vi "VI Server_GetClusterControlRefsAndMergeWithMainDataCluster.vi"(7 "Cluster.LabelArray":string[](array[string]), 8 "error in":errorcluster, 11 "VI Server Cluster":T1) -> (0 "error out":errorcluster, 1 "Cluster.ControRefs":refnum<vi>[](array[refnum]), 2 "Cluster.ControlLabels":string[](array[string]), 3 "VI Server Cluster.OUT":T1)   [LabVIEW 2020]
doc: "Retrieves multiple clusters' content labels and associated references and adds them to VI Server Cluster.\nIn addition it returns arrays of references and labels of the specified clusters.\n\nThis way these controls can be accessed via VI Server Tools.\nPlease keep in mind the labels should be unique in order to be properly identified."
uses:
  VI Server_TypeDefs/VI Server_RefsCluster.ctl
  VI Server Toolkit LV2013.lvlib
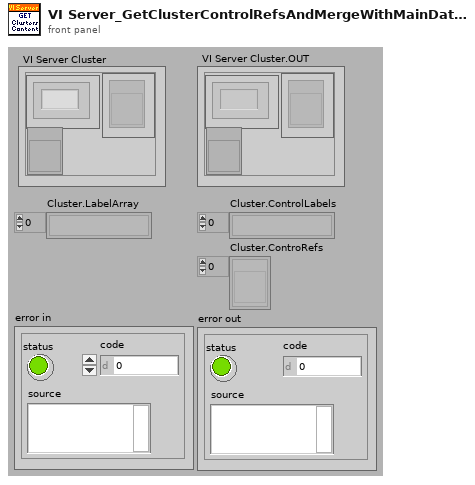
[diagram p1: front panel]
types:
  T1 = typedef "VI Server_RefsCluster.ctl" = cluster{"Labels":string[], "Refs":refnum<vi>[], "VI Ref":refnum<vi>}
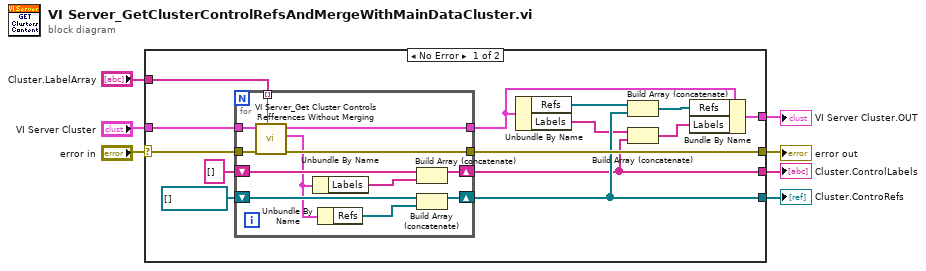
[diagram p0: block diagram]
diagram:
  n1 = case shown="No Error" "error in" {
    selector: "error in" -> [w16 w34]
    tunnel: [w11 _] -> w7
    tunnel: [w14 _] -> w6
    tunnel: "Cluster.LabelArray" -> [w19 _]
    tunnel: [w9 _] -> w4
    tunnel: "VI Server Cluster" -> [w18 _]
    tunnel: [w17 w34] -> w2
    frame No Error {
      n2 = for {
        tunnel: w16 -> [w33]
        tunnel: [w32] -> w17
        tunnel: w18 -> [w31]
        tunnel: [w30] -> w8
        tunnel: w19 -> [w29] mode=indexing
        shift-right: [w27] -> w11
        shift-left: string[] [] ("ClasterControlLabels") -> [w28]
        shift-right: [w25] -> w14
        shift-left: refnum<vi>[] [] ("ClasterControRefs") -> [w26]
        n3 = call "VI Server_Get Cluster Controls Refferences Without Merging.vi"("Cluster.Label"=w29, "error in"=w33, "VI Server Cluster"=w31) -> ("error out"=w32:errorcluster, "Cluster.VI Server Cluster"=w23:T1, "VI Server Cluster.DUP"=w30:T1)  [unwired: 6 in]
        n4 = Unbundle By Name(w23) -> ("Labels"=w24:string[])
        n5 = Unbundle By Name(w23) -> ("Refs"=w22:refnum<vi>[])
        n6 = Build Array (concatenate)(w28, w24) -> (w27:string[])
        n7 = Build Array (concatenate)(w26, w22) -> (w25:refnum<vi>[])
      }
      n8 = Unbundle By Name(w8) -> ("Refs"=w15:refnum<vi>[], "Labels"=w12:string[])
      n9 = Build Array (concatenate)(w15, w14) -> (w13:refnum<vi>[])
      n10 = Build Array (concatenate)(w12, w11) -> (w10:string[])
      n11 = Bundle By Name(cluster=w8, "Refs"=w13, "Labels"=w10) -> (w9:T1)
    }
    frame Error {
    }
  }
  "Cluster.ControlLabels" <- w7
  "Cluster.ControRefs" <- w6
  "VI Server Cluster.OUT" <- w4
  "error out" <- w2
